vi "LSX Get Switch Active.vi"(0 "lLSID":i32, 1 "plRA":i32, 5 "plXA":i32, 7 "plYA":i32, 9 "plZA":i32, 11 "error in (no error)":errorcluster) -> (3 "plRA out":i32, 4 "function return":i32, 6 "plXA out":i32, 8 "plYA out":i32, 10 "plZA out":i32, 15 "error out":errorcluster)   [LabVIEW 2016, in "Tango_DLL.lvlib"]
doc: "TANGOAPI int TANGOCALL LSX_GetSwitchActive (int lLSID, int *plXA, int *plYA, int *plZA, int *plRA);"
uses:
  Tango_DLL.lvlib
  2017/Microscope Control/Device Library/Stages/Marzhauser/SCAN IM 120 x 80/Tango DLL VIs/Tango_DLL.dll
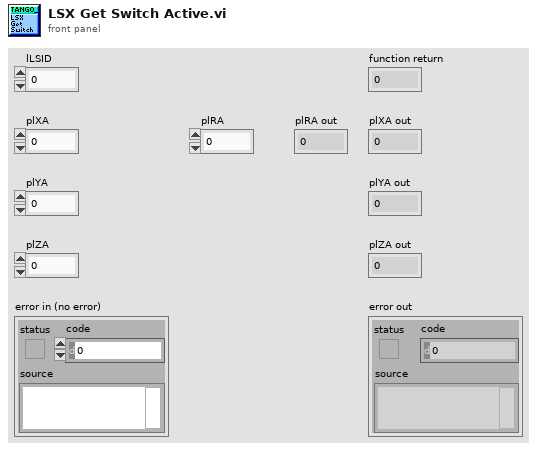
[diagram p1: front panel]
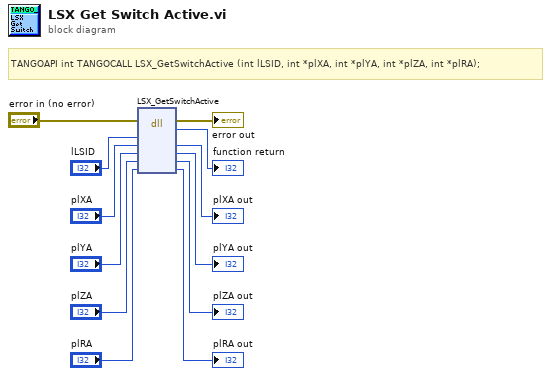
[diagram p0: block diagram]
diagram:
  # "TANGOAPI int TANGOCALL LSX_GetSwitchActive (int lLSID, int *plXA, int *plYA, int *plZA, int *plRA);"
  n1 = dll-call lib="C:/Users/4PiSMS/Documents/Microscope Control/2017/Microscope Control/Device Library/Stages/Marzhauser/SCAN IM 120 x 80/Tango DLL VIs/Tango_DLL.*" fn="LSX_GetSwitchActive"(error in="error in (no error)", "lLSID"="lLSID", "plXA"="plXA", "plYA"="plYA", "plZA"="plZA", "plRA"="plRA") -> (error out=→"error out":errorcluster, →"function return":i32, "plXA"=→"plXA out":i32, "plYA"=→"plYA out":i32, "plZA"=→"plZA out":i32, "plRA"=→"plRA out":i32)  [unwired: 3 in, 1 out]
